vi "ReadMediaPlayerRef.vi"(8 "Error In":errorcluster, 11 "reference in":refnum<class "Client.lvclass">) -> (0 "Error Out":errorcluster, 2 "MediaPlayerRef":refnum<class "MediaPlayer.lvclass">, 3 "reference out":refnum<class "Client.lvclass">)   [LabVIEW 2024, in "Client.lvclass"]
uses:
  Client.lvclass
  Receiver/MediaPlayer_class/MediaPlayer.lvclass
  Client.lvclass/Client.ctl
panel:
  # "Connector Pane"
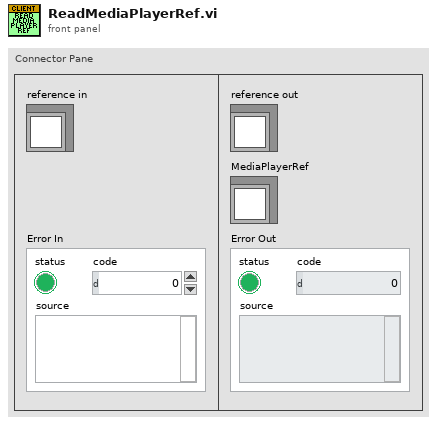
[diagram p1: front panel]
types:
  T1 = typedef "Client.lvclass/ObjectAttributes.ctl" = cluster{"RemoteControlRef":refnum<class "RemoteControl.lvclass">, "MediaPlayerRef":refnum<class "MediaPlayer.lvclass">}
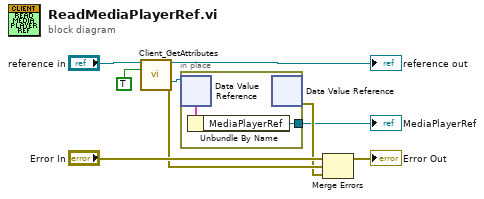
[diagram p0: block diagram]
diagram:
  n1 = call "Client_GetAttributes.vi"("reference in"="reference in", "OnlyGetDvrReference(False)"=TRUE) -> ("reference out"=→"reference out":refnum<class "Client.lvclass">, "DataRef"=w2:refnum<data-value>, "Error Out"=w8:errorcluster)  [unwired: 10 in, 1 out]
  n2 = in-place {
    in-place-border: [w11] -> w1
    n3 = in-place-dvr #1(w2) -> (w10:T1)  [unwired: 1 out]
    n4 = Unbundle By Name(w10) -> ("MediaPlayerRef"=w11:refnum<class "MediaPlayer.lvclass">)
    n5 = in-place-dvr #1() -> (w6:errorcluster)  [unwired: 1 in, 1 out]
  }
  "MediaPlayerRef" <- w1
  n6 = Merge Errors("Error In", w8, w6) -> (→"Error Out":errorcluster)
